vi "LWXPS_GetZone.vi"(1 "XPS Reference IN":refnum<k24>, 4 "LabVIEW error IN":errorcluster) -> (12 "XPS Reference OUT":refnum<k24>, 13 "LabVIEW error OUT":errorcluster, 14 "Returned error code":i32, 15 "X center in µm":dbl, 16 "Y center in µm":dbl, 17 "Radius in µm":dbl, 18 "Hysteresis in µm":dbl, 19 "XPS Error String":string)   [LabVIEW 2014]
uses:
  D:/XPSQ8_LabView_Library/Development/Source/Dll/Newport.XPS.CommandInterface.dll
  Dll/Newport.XPS.CommandInterface.dll
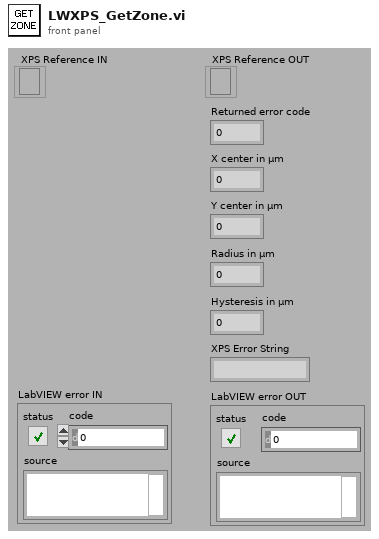
[diagram p1: front panel]
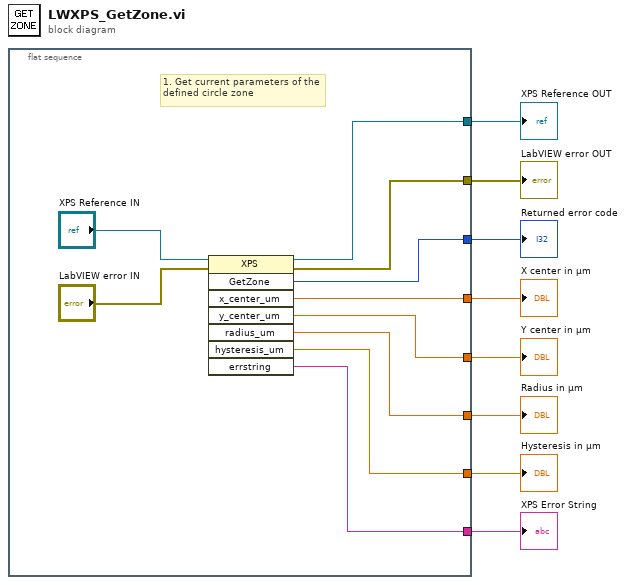
[diagram p0: block diagram]
diagram:
  n1 = flat-sequence {
    tunnel: [w13] -> w8
    tunnel: [w17] -> w7
    tunnel: [w15] -> w6
    tunnel: [w14] -> w3
    tunnel: [w12] -> w4
    tunnel: [w11] -> w2
    tunnel: [w10] -> w1
    tunnel: [w9] -> w5
    frame #0 {
      # "1. Get current parameters of the defined circle zone"
      n2 = invoke class="XPS" method="GetZone"(reference="XPS Reference IN", error in="LabVIEW error IN") -> (reference out=w13:refnum<k24>, error out=w17:errorcluster, "GetZone"=w15:i32, "x_center_um"=w12:dbl, "y_center_um"=w14:dbl, "radius_um"=w11:dbl, "hysteresis_um"=w10:dbl, "errstring"=w9:string)  [unwired: 6 in]
    }
  }
  "XPS Reference OUT" <- w8
  "LabVIEW error OUT" <- w7
  "Returned error code" <- w6
  "XPS Error String" <- w5
  "X center in µm" <- w4
  "Y center in µm" <- w3
  "Radius in µm" <- w2
  "Hysteresis in µm" <- w1
